vi "zadanie_1.vi"() -> ()   [LabVIEW 2020]
panel:
  out "Area (cm^2)":dbl
  in  "Radius (cm)":dbl(slide) scale=0.0..10.0
  out "Area (cm^2)":dbl
  in  "Base (cm)":dbl
  in  "Height (cm)":dbl
  # "Area of a Triangle"
  # "Area of a Circle"
  # "<---- Height ---->"
  # "r"
  # "<---- Base ---->"
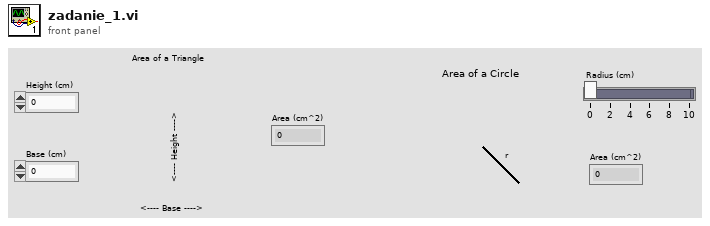
[diagram p1: front panel]
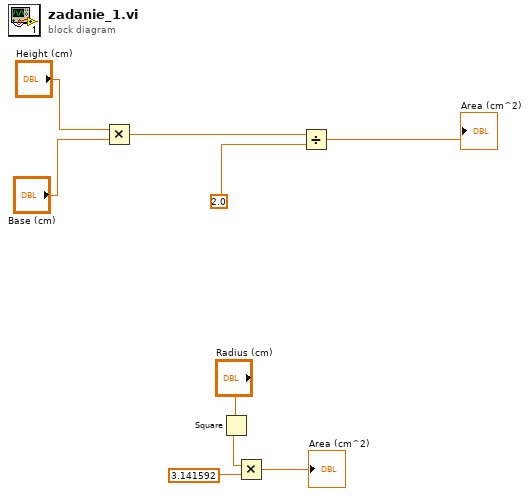
[diagram p0: block diagram]
diagram:
  n1 = Multiply(x="Height (cm)", y="Base (cm)") -> (x*y=w6:dbl)
  n2 = Square(x="Radius (cm)") -> (x^2=w3:dbl)
  n3 = Multiply(x=w3, y=3.141592) -> (x*y=→"Area (cm^2)":dbl)
  n4 = Divide(x=w6, y=2.0) -> (x/y=→"Area (cm^2)":dbl)
